vi "FisherPaykel Read Serial Command.vi"(7 "Debug":bool, 8 "Error In":errorcluster, 11 "VISA Refnum in":refnum<visa-resource-name>) -> (0 "Error Out":errorcluster, 2 "Serial Read Command":string, 3 "VISA Refnum out":refnum<visa-resource-name>)   [LabVIEW 2016]
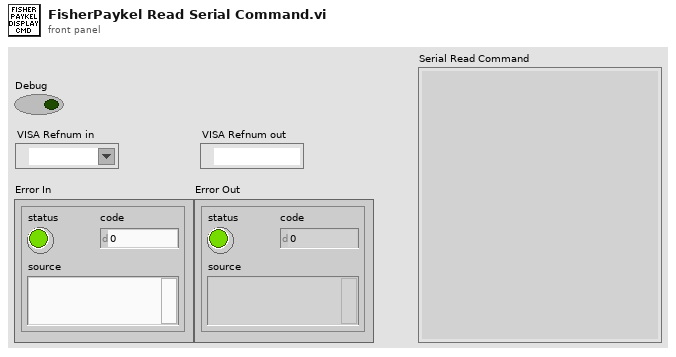
[diagram p1: front panel]
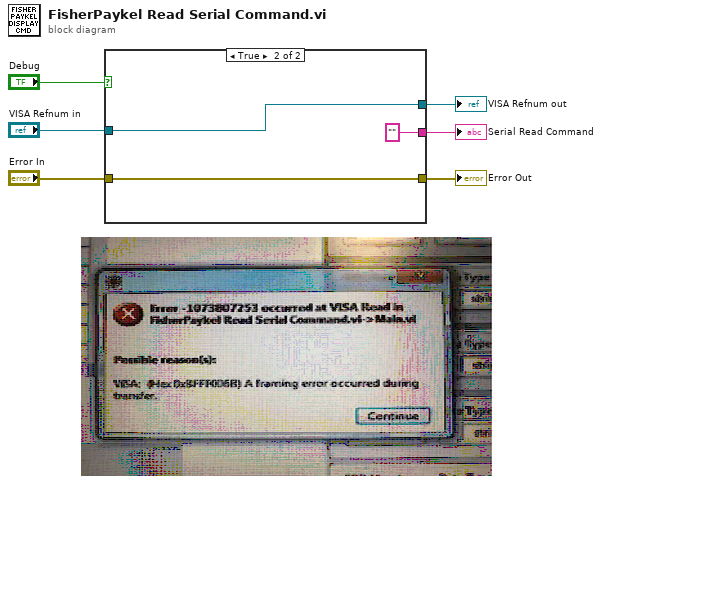
[diagram p0: block diagram]
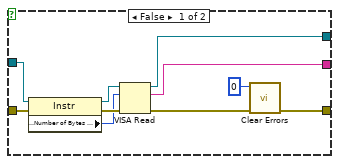
[diagram p2: hidden frame]
diagram:
  n1 = case shown="True" "Debug" {
    tunnel: [w15 "" ("read buffer")] -> w6
    tunnel: [w14 w19] -> w5
    tunnel: "VISA Refnum in" -> [w13 w19]
    tunnel: "Error In" -> [w11 w17]
    tunnel: [w8 w17] -> w2
    frame False {
      n2 = property class="Instr"(reference=w13, error in=w11) -> (reference out=w12:refnum<visa-resource-name>, error out=w16:errorcluster, "Serial Settings:Number of Bytes at Serial Port"=w10:u32)
      n3 = VISA Read(VISA resource name=w12, byte count=w10, error in (no error)=w16) -> (VISA resource name out=w14:refnum<visa-resource-name>, read buffer=w15:string, error out=w9:errorcluster)  [unwired: 1 out]
      n4 = call <vilib>:"Clear Errors.vi"("error in (no error)"=w9, "specific error code to clear (0: all)"=0) -> ("error out"=w8:errorcluster)  [unwired: 4 in, 1 out]
    }
    frame True {
    }
  }
  "Serial Read Command" <- w6
  "VISA Refnum out" <- w5
  "Error Out" <- w2
